vi "Save_templete_test.vi"() -> ()   [LabVIEW 2023]
uses:
  <vilib>/Utility/sysdir.llb/System Directory Type.ctl
  <vilib>/Utility/file.llb/Write Delimited Spreadsheet (string).vi
panel:
  out "참조 번호 출력":refnum<file>
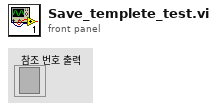
[diagram p1: front panel]
types:
  T1 = enum16{"open", "replace", "create", "open or create", "replace or create", "replace or create with confirmation"}
  T2 = typedef "System Directory Type.ctl" = i32
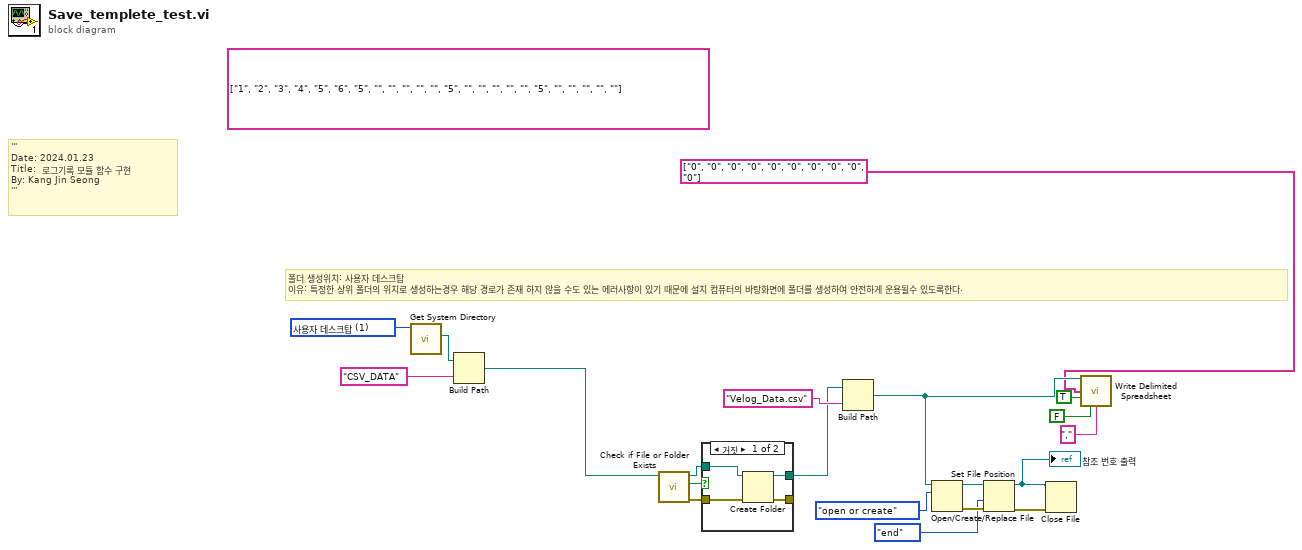
[diagram p0: block diagram]
diagram:
  (unwired) string[][] [["1", "2", "3", "4", "5", "6"], ["5", "", "", "", "", ""], ["5", "", "", "", "", ""], ["5", "", "", "", "", ""]]
  w14 = T2 1 items=["사용자 홈"=0, "사용자 데스크탑"=1, "사용자 문서"=2, "사용자 어플리케이션 데이터"=3, "사용자 환경"=4, "사용자 임시"=5, "퍼블릭 문서"=6, "퍼블릭 어플리케이션 데이터"=7, "퍼블릭 환경"=8, "퍼블릭 캐시"=13, "시스템 코어 라이브러리"=9, "시스템 설치된 라이브러리"=10, "어플리케이션 파일"=11, "부팅 볼륨 루트"=12] ("system directory type")
  # "폴더 생성위치: 사용자 데스크탑\n이유: 특정한 상위 폴더의 위치로 생성하는경우 해당 경로가 존재 하지 않을 수도 있는 에러사항이 있기 때문에 설치 컴퓨터의 바탕화면에 폴더를 생성하여 안전하게 운용될수 있도록한다."
  # "'''\nDate: 2024.01.23\nTitle:  로그기록 모듈 함수 구현\nBy: Kang Jin Seong\n'''"
  n1 = call <vilib>:"Get System Directory.vi"("system directory type"=w14) -> ("system directory"=w20:path)  [unwired: 10 in]
  n2 = Build Path(base path=w20, name or relative path="CSV_DATA") -> (appended path=w6:path)
  n3 = call <vilib>:"Check if File or Folder Exists.vi"("path"=w6) -> ("error out"=w17:errorcluster, "file or folder exists?"=w19:bool, "dup path"=w18:path)  [unwired: 8 in]
  n4 = case shown="거짓" w19 {
    tunnel: w18 -> [w24 w26]
    tunnel: w17 -> [w23 w25]
    tunnel: [w22 w26] -> w5
    tunnel: [w21 w25] -> _
    frame False {
      n5 = Create Folder(path (use dialog)=w24, error in=w23) -> (created path=w22:path, error out=w21:errorcluster)  [unwired: 1 in, 1 out]
    }
    frame True {
    }
  }
  n6 = Build Path(base path=w5, name or relative path="Velog_Data.csv") -> (appended path=w4:path)
  n7 = Open/Create/Replace File(file path (use dialog)=w4, operation (0:open)=T1."open or create" ("동작(0:open)")) -> (refnum out=w13:refnum<file>, error out=w12:errorcluster)  [unwired: 4 in, 1 out]
  n8 = Set File Position(refnum=w13, from (0:start)=enum16{"start", "end", "current"}."end" ("위치(0:start)"), error in=w12) -> (refnum out=w8:refnum<file>, error out=w9:errorcluster)  [unwired: 1 in]
  "참조 번호 출력" <- w8
  n9 = Close File(refnum=w8, error in=w9) -> ()  [unwired: 2 out]
  n10 = call-poly <vilib>:"Write Delimited Spreadsheet.vi"("file path (dialog if empty)"=w4, "1D data"=string[] ["0", "0", "0", "0", "0", "0", "0", "0", "0", "0"], "append to file? (new file:F)"=TRUE, "transpose? (no:F)"=FALSE, "delimiter (\\t)"="," ("delimiter (\\t)")) -> ()  [unwired: 9 in, 2 out]
